vi "YAML.NestedSection.vi"(2 "Section Key":string, 3 "Nested Section":string) -> (1 "String":string)   [LabVIEW 2016, in "Control Experiment.lvclass"]
uses:
  Control Experiment.lvclass
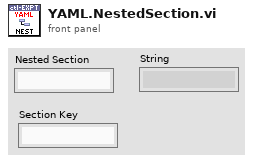
[diagram p1: front panel]
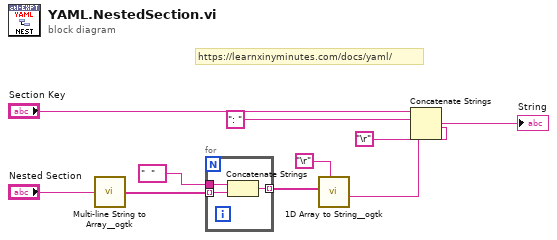
[diagram p0: block diagram]
diagram:
  # "https://learnxinyminutes.com/docs/yaml/"
  n1 = call <userlib>:"Multi-line String to Array__ogtk.vi"("string"="Nested Section") -> ("lines"=w4:string[])
  n2 = for {
    tunnel: w4 -> [w13] mode=indexing
    tunnel: "  " ("string") -> [w11]
    tunnel: [w12] -> w9 mode=indexing
    n3 = Concatenate Strings(w11, w13) -> (w12:string)
  }
  n4 = call <userlib>:"1D Array to String__ogtk.vi"("delimiter (Tab)"="\r", "Array of Strings"=w9) -> ("delimited string"=w7:string)  [unwired: 9 in]
  n5 = Concatenate Strings("Section Key", ": " ("string"), "\r", w7) -> (→"String":string)
